vi "Pause Logging.vi"(8 "error in (no error)":errorcluster, 11 "Data Logger Interface in":refnum<class "TDMS Data Logger Actor.lvclass">) -> (0 "error out":errorcluster, 3 "Data Logger Interface out":refnum<class "TDMS Data Logger Actor.lvclass">)   [LabVIEW 2024, in "TDMS Data Logger Actor.lvlib" / "TDMS Data Logger Actor.lvclass"]
uses:
  TDMS Data Logger Actor.lvclass
  C:/Program Files (x86)/National Instruments/LabVIEW 2024/vi.lib/ActorFramework/Actor/Actor.lvclass
  TDMS Data Logger Actor.lvclass/TDMS Data Logger Actor.ctl
  <vilib>/ActorFramework/Actor/Actor.lvclass/Actor.ctl
  <vilib>/ActorFramework/Message Enqueuer/Message Enqueuer.lvclass/Message Enqueuer.ctl
  <vilib>/ActorFramework/Message Enqueuer/Enqueue.vi
  Data Logger Actor Reply Interface/Data Logger Actor Reply Interface Messages/Logging Paused Msg/Logging Paused Msg.lvclass
  C:/Program Files (x86)/National Instruments/LabVIEW 2024/vi.lib/ActorFramework/Message/Message.lvclass
  <vilib>/ActorFramework/Message Priority Queue/Priority Enqueue.vi
  <vilib>/ActorFramework/Actor/Actor.lvclass
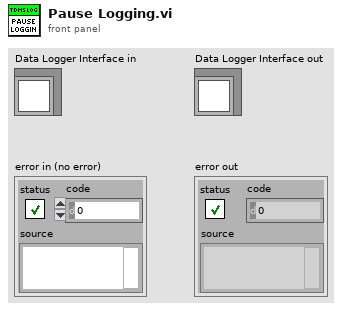
[diagram p1: front panel]
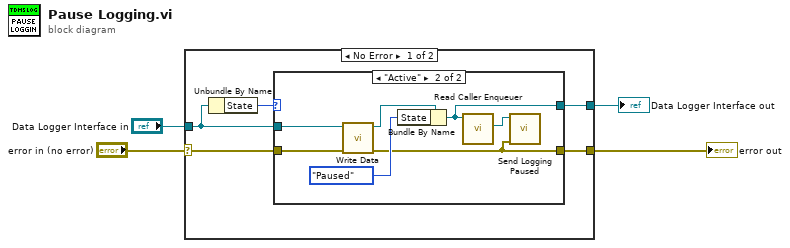
[diagram p0: block diagram]
diagram:
  n1 = case shown="No Error" "error in (no error)" {
    selector: "error in (no error)" -> [w6 w19]
    tunnel: "Data Logger Interface in" -> [w8 w20]
    tunnel: [w7 w20] -> w2
    tunnel: [w5 w19] -> w1
    frame No Error {
      n2 = Unbundle By Name(w8) -> ("State"=w9:enum16{"Idle", "Active", "Paused"})
      n3 = case shown="\"Active\"" w9 {
        tunnel: w8 -> [w10 w15]
        tunnel: [w10 w17] -> w7
        tunnel: w6 -> [w11 w13]
        tunnel: [w11 w12] -> w5
        frame "Idle", "Paused" {
        }
        frame "Active" {
          n4 = call-dynamic "Write Data.vi"("error in (no error)"=w13, "TDMS Data Logger Actor in"=w15) -> ("error out"=w12:errorcluster, "TDMS Data Logger Actor out"=w14:refnum<class "TDMS Data Logger Actor.lvclass">)  [unwired: 8 in]
          n5 = Bundle By Name(cluster=w14, "State"=enum16{"Idle", "Active", "Paused"}."Paused") -> (w17:refnum<class "TDMS Data Logger Actor.lvclass">)
          n6 = call <vilib>:"Read Caller Enqueuer.vi"("Actor"=w17) -> ("Caller Enqueuer"=w16:refnum<class "Message Enqueuer.lvclass">)  [unwired: 10 in]
          n7 = call "Send Logging Paused.vi"("error in (no error)"=w12, "Message Enqueuer"=w16) -> ()  [unwired: 8 in, 2 out]
        }
      }
    }
    frame Error {
    }
  }
  "error out" <- w1
  "Data Logger Interface out" <- w2
